vi "Get Time Unit.vi"(0 "VISA resource name":refnum<visa-resource-name>, 11 "error in (no error)":errorcluster) -> (4 "VISA resource name out":refnum<visa-resource-name>, 6 "Time Unit":enum16{"Seconds", "Minutes", "Hours"}(ring), 15 "error out":errorcluster)   [LabVIEW 2016, in "APT 300XAC Series.lvlib"]
doc: "Gets the time unit currently set in the power source instrument.\n\nNote : Time unit behaves different in the following firmware version\n\nProgram Mode : it is a Step Parameter (Can be configured in every step individually).\nManual Mode : Not Supported\nDC Mode : Not Supported"
uses:
  APT 300XAC Series.lvlib
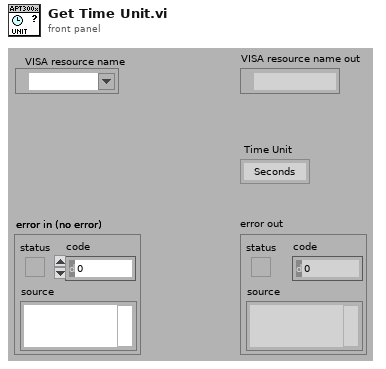
[diagram p1: front panel]
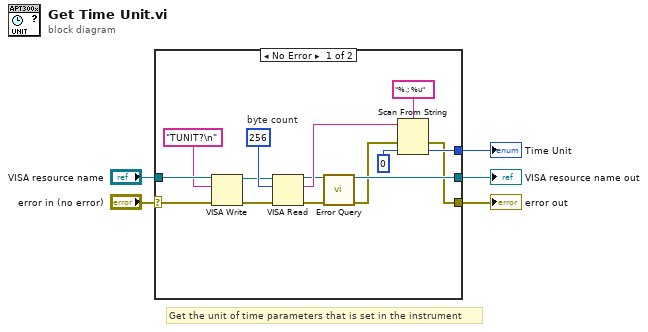
[diagram p0: block diagram]
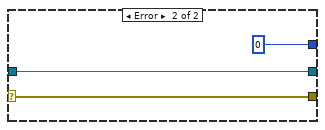
[diagram p2: hidden frame]
diagram:
  # "Get the unit of time parameters that is set in the instrument"
  n1 = case shown="No Error" "error in (no error)" {
    selector: "error in (no error)" -> [w19 w23]
    tunnel: "VISA resource name" -> [w20 w22]
    tunnel: [w11 w22] -> w4
    tunnel: [w6 w23] -> w3
    tunnel: [w13 u16 0] -> w1
    frame No Error {
      w16 = u32 256  # byte count
      n2 = VISA Write(VISA resource name=w20, write buffer="TUNIT?\n", error in (no error)=w19) -> (VISA resource name out=w14:refnum<visa-resource-name>, error out=w15:errorcluster)  [unwired: 1 out]
      n3 = VISA Read(VISA resource name=w14, byte count=w16, error in (no error)=w15) -> (VISA resource name out=w10:refnum<visa-resource-name>, read buffer=w12:string, error out=w9:errorcluster)  [unwired: 1 out]
      n4 = call "Error Query.vi"("VISA resource name"=w10, "error in (no error)"=w9) -> ("VISA resource name out"=w11:refnum<visa-resource-name>, "error out"=w7:errorcluster)  [unwired: 10 in, 2 out]
      n5 = Scan From String(format string="%.; %u" ("Format String"), input string=w12, error in=w7, default 1=0 ("default value 1")) -> (error out=w6:errorcluster, output 1=w13:i32)  [unwired: 1 in, 2 out]
    }
    frame Error {
    }
  }
  "error out" <- w3
  "VISA resource name out" <- w4
  "Time Unit" <- w1
